vi "external_api_init.vi"(8 "error in (no error)":errorcluster, 11 "Port (5555)":i32=5555) -> (0 "error out":errorcluster, 2 "socket out":refnum<class "zmq_socket.lvclass">, 3 "zmq_context out":refnum<class "zmq_context.lvclass">)   [LabVIEW 2020]
uses:
  <vilib>/addons/zeromq/zmq_socket.lvclass
  <vilib>/addons/zeromq/zmq_context.lvclass
  <vilib>/addons/zeromq/socket_type.ctl
  src/labview/global API.vi
  <vilib>/addons/zeromq/zeromq.lvlib
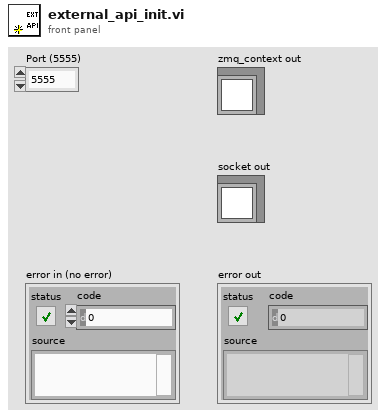
[diagram p1: front panel]
types:
  T1 = typedef "zeromq.lvlib/socket_type.ctl" = enum8{"ZMQ_PAIR", "ZMQ_PUB", "ZMQ_SUB", "ZMQ_REQ", "ZMQ_REP", "ZMQ_DEALER", "ZMQ_ROUTER", "ZMQ_PULL", "ZMQ_PUSH", "ZMQ_XPUB", "ZMQ_XSUB", "ZMQ_STREAM", "ZMQ_SERVER", "ZMQ_CLIENT", "ZMQ_RADIO", "ZMQ_DISH", "ZMQ_GATHER", "ZMQ_SCATTER", "ZMQ_DGRAM"}
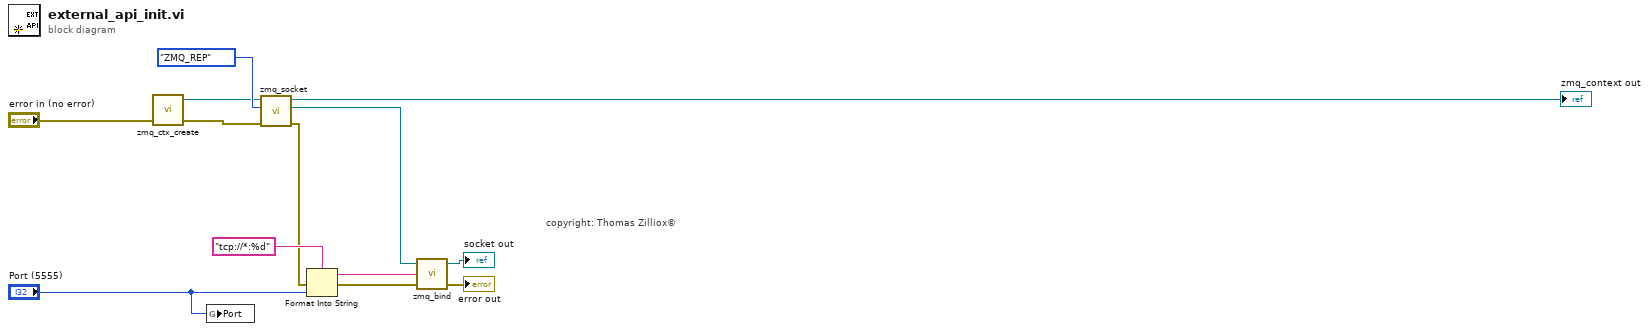
[diagram p0: block diagram]
diagram:
  # "copyright: Thomas Zilliox©"
  n1 = call <vilib>:"zmq_ctx_create.vi"("error in"="error in (no error)") -> ("error out"=w4:errorcluster, "context out"=w3:refnum<class "zmq_context.lvclass">)  [unwired: 3 in]
  n2 = global write "global API.vi" "Port"("Port (5555)") -> ()
  n3 = call <vilib>:"zmq_socket.vi"("error in"=w4, "socket type"=socket_type."ZMQ_REP", "context in"=w3) -> ("error out"=w8:errorcluster, "socket out"=w7:refnum<class "zmq_socket.lvclass">, "context out"=→"zmq_context out":refnum<class "zmq_context.lvclass">)  [unwired: 2 in]
  n4 = Format Into String(format string="tcp://*:%d" ("endpoint"), error in=w8, "Port (5555)") -> (resulting string=w12:string, error out=w11:errorcluster)  [unwired: 1 in]
  n5 = call <vilib>:"zmq_bind.vi"("error in"=w11, "endpoint"=w12, "socket in"=w7) -> ("error out"=→"error out":errorcluster, "socket out"=→"socket out":refnum<class "zmq_socket.lvclass">)  [unwired: 1 in]
